vi "SystemEinstellungenV2DateiLesen.vi"(6 "Dateiname":string, 8 "Fehler (Eingang)":errorcluster, 9 "[Optionen]":string, 10 "[AnalysatorenDefinition]":string, 11 "[GasteilerDefinition]":string) -> (0 "Fehler (Ausgang)":errorcluster, 1 "[Optionen]":string[][](array[string]), 2 "[AnalysatorenDefinition]":string[][](array[string]), 3 "[GasteilerDefinition]":string[][](array[string]))   [LabVIEW 2020, in "System Einstellungen V2.lvlib"]
uses:
  System Einstellungen V2.lvlib
  Allgemein/allgemeine Sub-VIs.lvlib
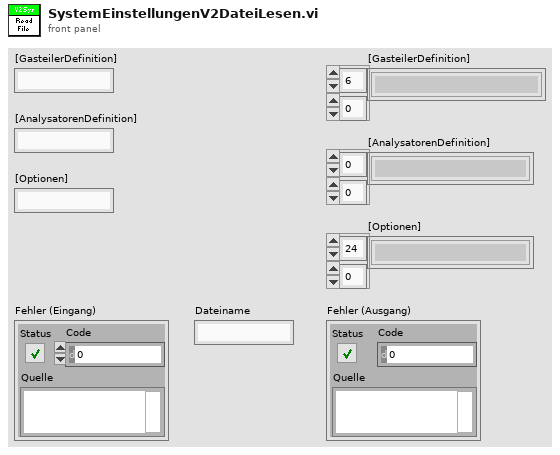
[diagram p1: front panel]
types:
  T1 = enum16{"open", "replace", "create", "open or create", "replace or create", "replace or create with confirmation"}
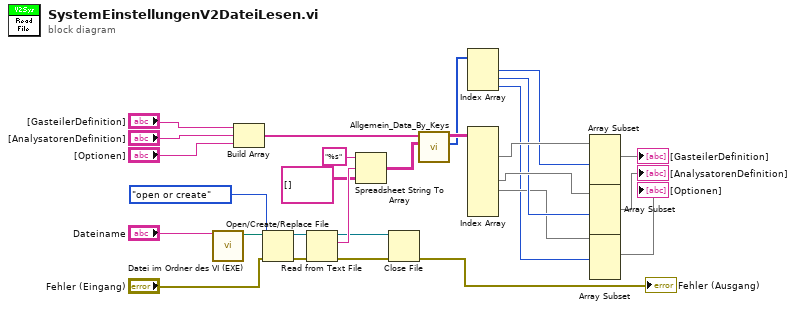
[diagram p0: block diagram]
diagram:
  n1 = call "Datei im Ordner des VI (EXE).vi"("Dateiname"="Dateiname") -> ("Dateipfad im Ordner des Haupt-VIs"=w17:path)  [unwired: 8 in, 2 out]
  n2 = Build Array("[GasteilerDefinition]", "[AnalysatorenDefinition]", "[Optionen]") -> (w15:string[])
  n3 = Open/Create/Replace File(file path (use dialog)=w17, error in="Fehler (Eingang)", operation (0:open)=T1."open or create" ("Operation (0:open)")) -> (refnum out=w19:refnum<file>, error out=w18:errorcluster)  [unwired: 3 in, 1 out]
  n4 = Read from Text File(file (use dialog)=w19, error in=w18) -> (refnum out=w20:refnum<file>, text=w26:string, error out=w21:errorcluster)  [unwired: 2 in, 1 out]
  n5 = Spreadsheet String To Array(format string="%s" ("Format-String"), spreadsheet string=w26, array type (2D Dbl)=string[][] [] ("String")) -> (array=w28:string[][])  [unwired: 1 in]
  n6 = Close File(refnum=w20, error in=w21) -> (error out=→"Fehler (Ausgang)":errorcluster)  [unwired: 1 out]
  n7 = call "Allgemein_Data_By_Keys.vi"("String"=w28, "Keys (Eingang)"=w15) -> ("Length Array  (Ausgang)"=w8:i32[], "Array (Ausgang)"=w11:string[][][])  [unwired: 8 in]
  n8 = Index Array(array=w8) -> (element #1=w7:i32, element #2=w4:i32, element #3=w1:i32)  [unwired: 3 in]
  n9 = Index Array(array=w11) -> (element #1=w9:string[][], element #2=w6:string[][], element #3=w3:string[][])  [unwired: 9 in]
  n10 = Array Subset(array=w9, length (row)=w7) -> (→"[GasteilerDefinition]":string[][])  [unwired: 3 in]
  n11 = Array Subset(array=w6, length (row)=w4) -> (→"[AnalysatorenDefinition]":string[][])  [unwired: 3 in]
  n12 = Array Subset(array=w3, length (row)=w1) -> (→"[Optionen]":string[][])  [unwired: 3 in]
